vi "Shutdown.vi"(8 "error in (no error)":errorcluster, 11 "MB in":refnum<class "Master CR.lvclass">) -> (0 "error out":errorcluster)   [LabVIEW 2021, in "Master CR.lvclass"]
doc: "Closes and destroys a Modbus master instance."
uses:
  Master CR.lvclass
  Master CR.lvclass/Master CR.ctl
  Modbus_v121c/Data Model/Device Data Model.lvclass
  Param/Param.lvclass
  Modbus_v121c/Network Protocol/Network Protocol.lvclass
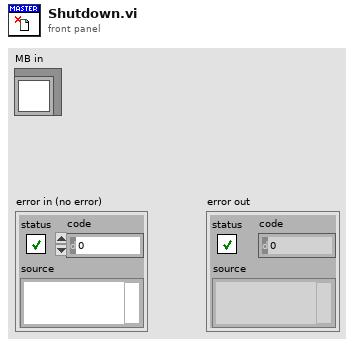
[diagram p1: front panel]
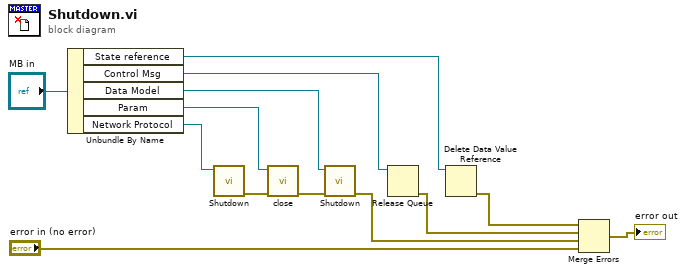
[diagram p0: block diagram]
diagram:
  n1 = Unbundle By Name("MB in") -> ("State reference"=w13:refnum<data-value>, "Control Msg"=w10:refnum<queue>, "Data Model"=w5:refnum<class "Device Data Model.lvclass">, "Param"=w3:refnum<class "Param.lvclass">, "Network Protocol"=w2:refnum<class "Network Protocol.lvclass">)
  n2 = call-dynamic "Shutdown.vi"("Network Protocol in"=w2) -> ("error out"=w1:errorcluster)  [unwired: 10 in]
  n3 = call-dynamic "close.vi"("error in"=w1, "MBParam in"=w3) -> ("error out"=w7:errorcluster)  [unwired: 9 in]
  n4 = call-dynamic "Shutdown.vi"("error in"=w7, "device data model in"=w5) -> ("error out"=w6:errorcluster)  [unwired: 9 in]
  n5 = Release Queue(queue=w10) -> (error out=w8:errorcluster)  [unwired: 2 in, 2 out]
  n6 = Delete Data Value Reference(data value reference=w13) -> (error out=w11:errorcluster)  [unwired: 1 in, 1 out]
  n7 = Merge Errors(w11, w8, w6, "error in (no error)") -> (→"error out":errorcluster)
